vi "SendDataEvent.vi"(6 "properties":T1[](array[typedef]), 7 "block":i32, 8 "error in (no error)":errorcluster, 9 "stream id":string, 10 "event reference":T2, 11 "Qbus in":refnum<class "Qbus.lvclass">) -> (0 "error out":errorcluster, 3 "Qbus out":refnum<class "Qbus.lvclass">)   [LabVIEW 2017, in "ServerComm.lvlib"]
doc: "Sends the data event to the server."
uses:
  <vilib>/addons/InsightCM/Devices/Shared/Common/ServerComm/ServerComm.lvlib
  <vilib>/addons/Qbus/Qbus.lvclass
  <vilib>/addons/InsightCM/Devices/Shared/Common/DataEvent/controls/EventReference.ctl
  <vilib>/addons/InsightCM/Devices/Shared/Common/DataEvent/controls/Event.ctl
  <vilib>/addons/InsightCM/MessageBus/Base/controls/DataEvent.ctl
  <vilib>/addons/InsightCM/MessageBus/Base/controls/KeyValuePair.ctl
  <vilib>/addons/InsightCM/Devices/Shared/Common/DataEvent/controls/DataSet.ctl
  <vilib>/addons/InsightCM/MessageBus/Base/controls/DataSetMetadata.ctl
  <vilib>/addons/InsightCM/MessageBus/Base/controls/TrendPoint.ctl
  <vilib>/addons/InsightCM/MessageBus/Base/controls/TrendAlarmUpdate.ctl
  <vilib>/addons/InsightCM/MessageBus/Base/controls/TrendAlarmTransition.ctl
  <vilib>/addons/InsightCM/Devices/Shared/Common/ServerComm/controls/SendDataEvent.ctl
  <vilib>/addons/InsightCM/Devices/Shared/Common/DataEvent/DataEvent.lvlib
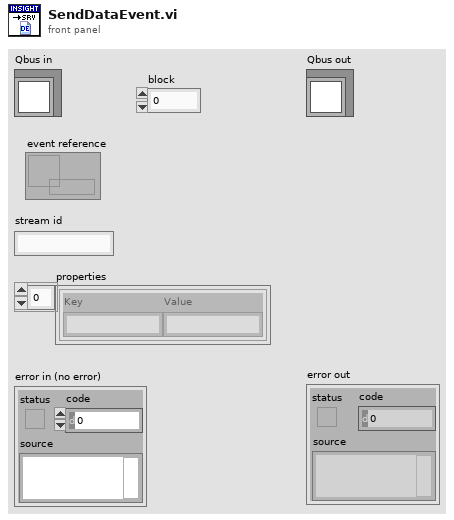
[diagram p1: front panel]
types:
  T1 = typedef "KeyValuePair.ctl" = cluster{"Key":string, "Value":string}
  T2 = typedef "DataEvent.lvlib/EventReference.ctl" = refnum<data-value>
  T3 = typedef "ServerComm.lvlib/SendDataEvent.ctl" = cluster{"event reference":T2, "StreamId":string, "Block":i32, "Properties":T1[]}
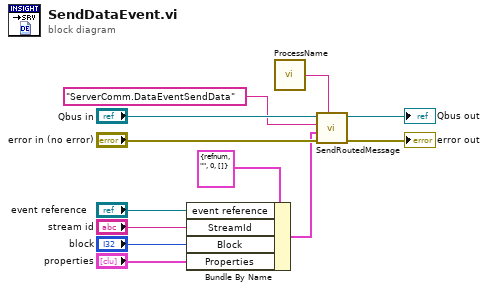
[diagram p0: block diagram]
diagram:
  n1 = Bundle By Name(cluster=T3 {"event reference"=refnum, "StreamId"="", "Block"=0, "Properties"=[]} ("Body"), "event reference"="event reference", "StreamId"="stream id", "Block"="block", "Properties"="properties") -> (w5:T3)
  n2 = call <vilib>:"ProcessName.vi"() -> ("process name"=w9:string)  [unwired: 5 in]
  n3 = call <vilib>:"SendRoutedMessage.vi"("listener process"=w9, "error in (no error)"="error in (no error)", "message value"=w5, "message name"="ServerComm.DataEventSendData", "Qbus in"="Qbus in") -> ("error in (no error)"=→"error out":errorcluster, "Qbus out"=→"Qbus out":refnum<class "Qbus.lvclass">)  [unwired: 5 in]
